vi "SetDelay2.vi"(8 "Mixer freq [MHz]":dbl, 9 "Output delay delta":dbl, 10 "Output delay":dbl, 11 "FPGA ref":T1) -> (3 "FPGA ref out":T1)   [LabVIEW 2013]
uses:
  controls/settingsFPGAref.ctl
  FPGA/fpga_settings.ctl
  <vilib>/rvi/interface/common/niFpgaWaitOnOcc.vi
  <vilib>/Utility/error.llb/Error Cluster From Error Code.vi
  <vilib>/rvi/errors/niLvFpgaAdjustHostInterfaceError.vi
  <vilib>/rvi/FXPMathLib/FxpInterpret/XNode/nifxpmath_Interpret.xnode
  <vilib>/rvi/interface/nirviReadWriteControl/nirviReadWriteControl.xnode
  NiFpgaLv.dll
  <vilib>/rvi/interface/Simulation/niFpgaSimulationCallBeginRW.vi
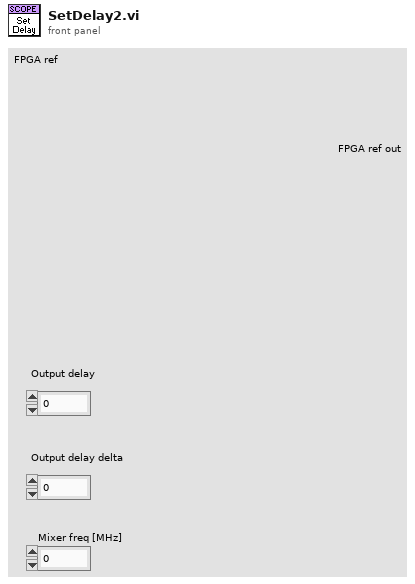
[diagram p1: front panel]
types:
  T1 = typedef "settingsFPGAref.ctl" = refnum<k20>
  T2 = typedef "fpga_settings.ctl" = enum16{"Feedback Enable", "New FIR coeffs", "FIR shift", "Enable filter", "Set Downsample", "Downsample", "CIC Gain", "Record length", "Trigger samples", "Quiet time", "a_am", "b_am", "Use fixed delay", "fixed sin_fi", "fixed cos_fi", "Ki*Tau", "Kp", "Kd_Tau", "Fi_start", "Fi_delta", "DC_offs 0", "DC_offs 1", "DC_offs 2", "DC_offs 3", "Ki*Tau am", "Kp am", "Kd_Tau am", "Feedback AM", "Trigger delay", "Feedback delay", "Setpoint enable", "Beam enable", "Samples to acquire"}
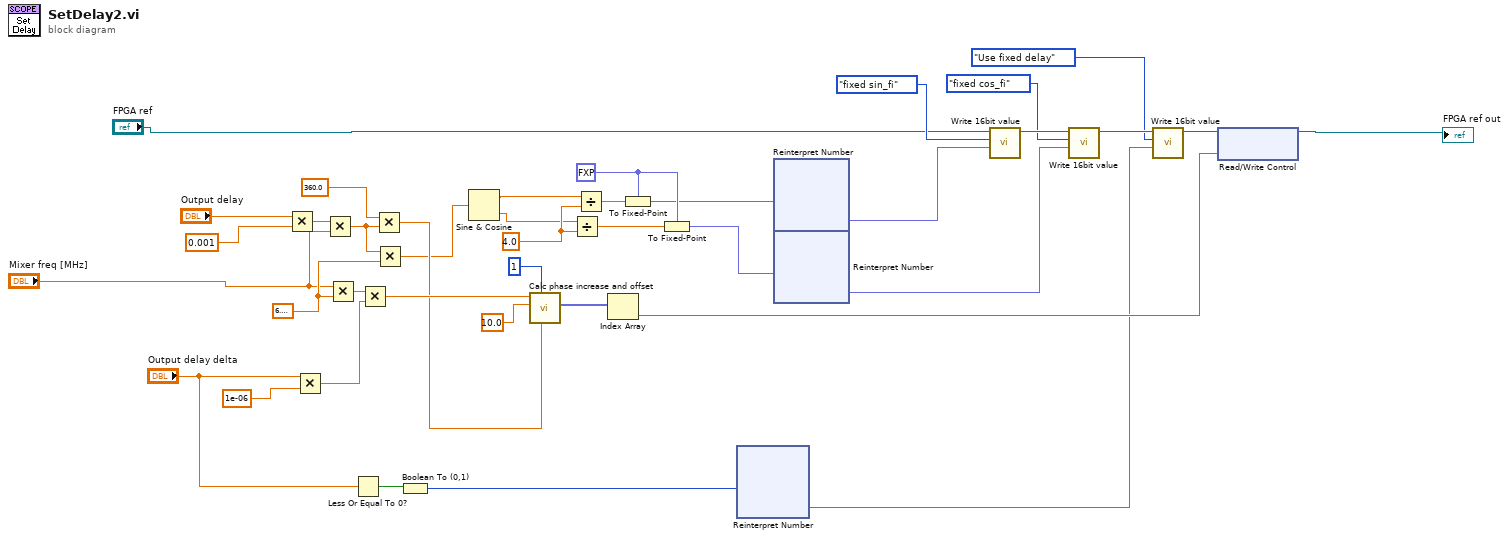
[diagram p0: block diagram]
diagram:
  w21 = 4.0 ("y")
  w22 = fxp<+/-,16,0> 0.0 ("fixed sin fi")
  w25 = 6.283185307179586
  n1 = Multiply(x="Output delay", y=0.001) -> (x*y=w31:dbl)
  n2 = Multiply(x="Output delay delta", y=1e-06) -> (x*y=w32:dbl)
  n3 = Multiply(x=w31, y="Mixer freq [MHz]") -> (x*y=w26:dbl)
  n4 = Multiply(x="Mixer freq [MHz]", y=w25) -> (x*y=w37:dbl)
  n5 = Less Or Equal To 0?(x="Output delay delta") -> (x <= 0?=w12:bool)
  n6 = Multiply(x=w37, y=w32) -> (x*y=w36:dbl)
  n7 = Multiply(x=360.0, y=w26) -> (x*y=w29:dbl)
  n8 = Multiply(x=w26, y=w25) -> (x*y=w24:dbl)
  n9 = Boolean To (0,1)(Boolean=w12) -> (0, 1=w11:i16)
  n10 = Sine & Cosine(0:w24) -> (1:w20:dbl, 2:w17:dbl)
  n11 = call "Calc phase increase and offset.vi"("Phase offset (deg)"=w29, "# of DDS"=1, "fclk (MHz)"=10.0, "f_generated (MHz)"=w36) -> ("Phase out"=w28:fxp<+,64,64>[])  [unwired: 5 in, 2 out]
  n12 = Divide(x=w17, y=w21) -> (x/y=w18:dbl)
  n13 = Divide(x=w20, y=w21) -> (x/y=w19:dbl)
  n14 = Index Array(array=w28) -> (element=w23:fxp<+,64,64>)  [unwired: 1 in]
  n15 = To Fixed-Point(fixed-point type=w22, number=w19) -> (fixed-point=w14:fxp<+/-,16,0>)
  n16 = To Fixed-Point(fixed-point type=w22, number=w18) -> (fixed-point=w13:fxp<+/-,16,0>)
  n17 = xnode "Reinterpret Number"("x"=w11) -> ("y"=w6:fxp<+,16,16>)
  n18 = xnode "Reinterpret Number"("x"=w14) -> ("y"=w15:fxp<+,16,16>)
  n19 = xnode "Reinterpret Number"("x"=w13) -> ("y"=w7:fxp<+,16,16>)
  n20 = call "Write 16bit value.vi"("value"=w15, "FPGA Setting"=fpga_settings."fixed sin_fi", "FPGA ref"="FPGA ref") -> ("FPGA ref out"=w10:T1)  [unwired: 7 in, 1 out]
  n21 = call "Write 16bit value.vi"("value"=w7, "FPGA Setting"=fpga_settings."fixed cos_fi", "FPGA ref"=w10) -> ("FPGA ref out"=w9:T1)  [unwired: 7 in, 1 out]
  n22 = call "Write 16bit value.vi"("value"=w6, "FPGA Setting"=fpga_settings."Use fixed delay", "FPGA ref"=w9) -> ("FPGA ref out"=w8:T1)  [unwired: 7 in, 1 out]
  n23 = xnode "Read/Write Control"("FPGA VI Reference In"=w8, "delay phase"=w23) -> ("FPGA VI Reference Out"=→"FPGA ref out":T1)  [unwired: 1 in, 1 out]
